vi "Report config errors.vi"(6 "SLSC Dynamic Inputs":T1[](array[typedef]), 8 "error in (no error)":errorcluster, 11 "Data Value Reference in":refnum<data-value>) -> (0 "error out":errorcluster)   [LabVIEW 2019, in "SLSC-12201 DIO Engine.lvlib"]
uses:
  SLSC-12201 DIO Engine.lvlib
  Shared/SLSC Dynamic Channel.ctl
  Shared/SLSC Dynamic Channel Type.ctl
  <vilib>/NI/NIVS Inline Async API/_Data Access Engine/Access Type Classes/Write/Write.lvclass
  <vilib>/NI/NIVS Inline Async API/_Data Access Engine/Access Type Classes/Write/Write.lvclass/Write.ctl
  <vilib>/NI/NIVS Inline Async API/_Data Access Engine/Data Access Engine/Methods/Write.Data.vi
  <vilib>/NI/NIVS Inline Async API/_Data Access Engine/Access Type Classes/Write/Write.ProcessData.vi
  <vilib>/NI/NIVS Inline Async API/_Data Access Engine/Access Type Classes/Write/Write.Buffer.vi
  <vilib>/NI/NIVS Inline Async API/_Data Access Engine/Access Type Classes/Write/Write.Commit.vi
  <vilib>/NI/NIVS Inline Async API/_Data Access Engine/Data Access Engine/Data Access Engine.lvclass
  Shared/SLSC-12201 DIO Shared.lvlib
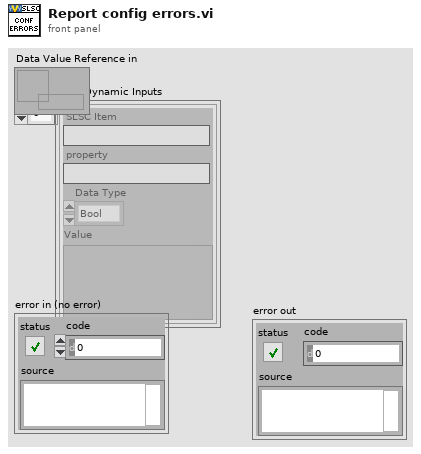
[diagram p1: front panel]
types:
  T1 = typedef "SLSC-12201 DIO Shared.lvlib/SLSC Dynamic Channel.ctl" = cluster{"SLSC Item":string, "property":string, "Data Type":T2, "Value":variant}
  T2 = typedef "SLSC-12201 DIO Shared.lvlib/SLSC Dynamic Channel Type.ctl" = enum16{"Bool", "Double", "I32", "I64", "String", "U32", "U64", "EnumI32"}
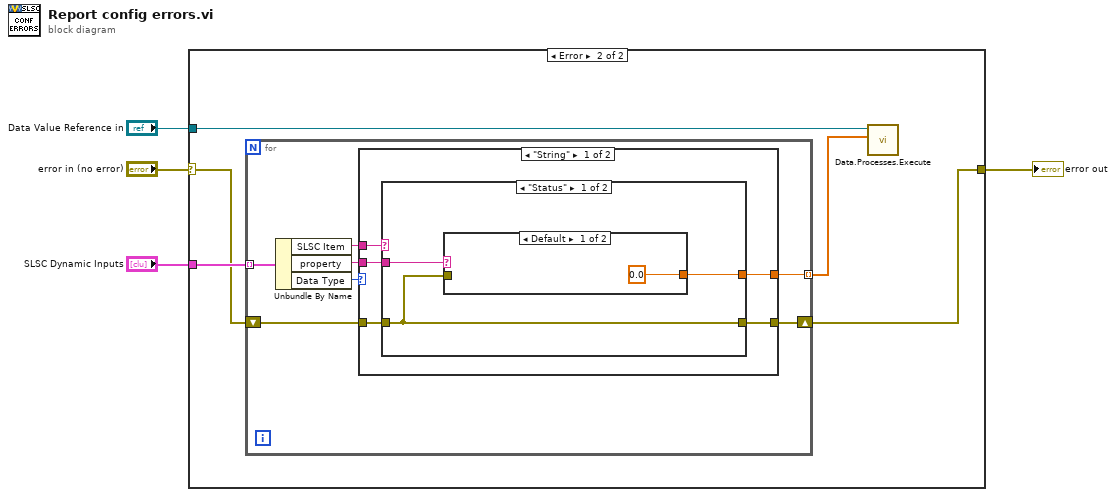
[diagram p0: block diagram]
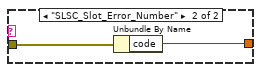
[diagram p3: hidden frame]
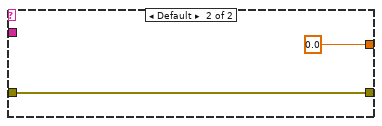
[diagram p4: hidden frame]
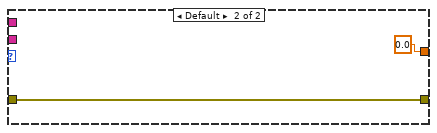
[diagram p5: hidden frame]
diagram:
  n1 = case shown="Error" "error in (no error)" {
    selector: "error in (no error)" -> [w5 w8]
    tunnel: "Data Value Reference in" -> [_ w10]
    tunnel: "SLSC Dynamic Inputs" -> [_ w9]
    tunnel: [w5 w6] -> w1
    frame No Error {
    }
    frame Error {
      n2 = for {
        tunnel: w9 -> [w17] mode=indexing
        tunnel: [w12] -> w7 mode=indexing
        shift-right: [w11] -> w6
        shift-left: w8 -> [w13]
        n3 = Unbundle By Name(w17) -> ("SLSC Item"=w14:string, "property"=w15:string, "Data Type"=w16:T2)
        n4 = case shown="\"String\"" w16 {
          tunnel: w15 -> [w22 _]
          tunnel: w14 -> [w19 _]
          tunnel: w13 -> [w21 w31]
          tunnel: [w20 0.0 ("LoopDuration(ms)")] -> w12
          tunnel: [w18 w31] -> w11
          frame "String" {
            n5 = case shown="\"Status\"" w19 {
              tunnel: w22 -> [w23 _]
              tunnel: w21 -> [w24 w29]
              tunnel: [w24 w29] -> w18
              tunnel: [w25 0.0 ("LoopDuration(ms)")] -> w20
              frame "Status" {
                n6 = case shown="Default" w23 {
                  tunnel: [0.0 ("LoopDuration(ms)") w27] -> w25
                  tunnel: w24 -> [_ w28]
                  frame Default {
                  }
                  frame "SLSC_Slot_Error_Number" {
                    n7 = Unbundle By Name(w28) -> ("code"=w27:i32)
                  }
                }
              }
              frame Default {
              }
            }
          }
          frame Default {
          }
        }
      }
      n8 = call-poly <vilib>:"Data.Processes.Execute.vi"("Values"=w7, "Ref"=w10) -> ()  [unwired: 9 in, 1 out]
    }
  }
  "error out" <- w1
